vi "DAQ_connect.vi"(10 "thermocouple type":i32(ring)=10073 items=["J"=10072, "K"=10073, "N"=10077, "R"=10082, "S"=10085, "T"=10086, "B"=10047, "E"=10055], 11 "Array":tag[](array[tag])=["Mod2/ai1", "Mod2/ai2"]) -> (0 "error out":errorcluster, 3 "Refnum out":refnum<k21>)   [LabVIEW 2021, in "DAQ_Termopares.lvlib"]
uses:
  DAQ_Termopares.lvlib
  <vilib>/DAQmx/create/channels.llb/DAQmx Create Channel (AI-Temperature-Thermocouple).vi
panel:
  out "Array 2":errorcluster[](array[cluster])
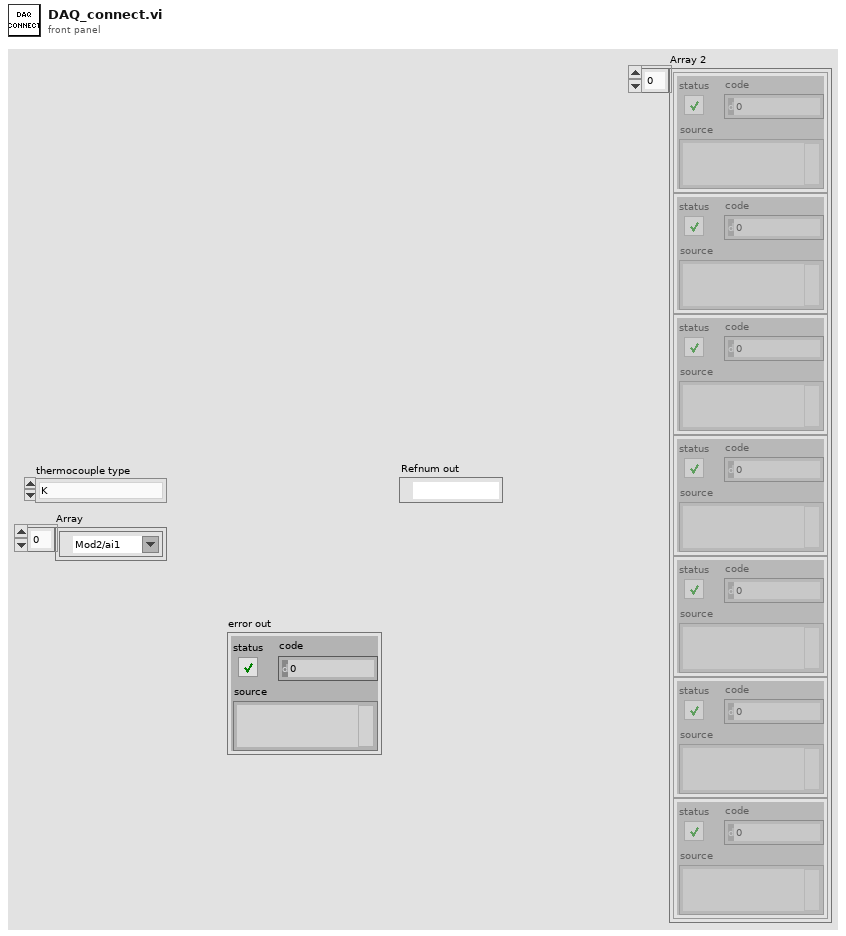
[diagram p1: front panel]
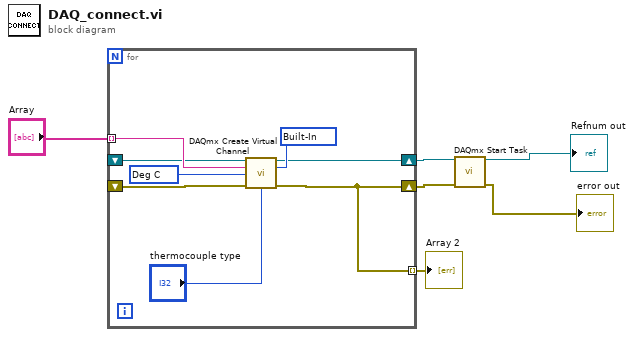
[diagram p0: block diagram]
diagram:
  n1 = for {
    tunnel: "Array" -> [w12] mode=indexing
    shift-right: [w7] -> w6
    shift-left: _ -> [w9]
    shift-right: [w11] -> w5
    shift-left: _ -> [w10]
    tunnel: [w7] -> w1 mode=indexing
    w14 = 10200 items=["Built-In"=10200, "Constant Value"=10116, "Channel"=10113] ("cjc source")
    w13 = 10143 items=["Deg C"=10143, "Deg F"=10144, "Kelvins"=10325, "Deg R"=10145, "From Custom Scale"=10065] ("units")
    n2 = call-poly <vilib>:"DAQmx Create Virtual Channel.vi"("task in"=w10, "physical channels"=w12, "cjc source"=w14, "units"=w13, "error in"=w9, "thermocouple type"="thermocouple type") -> ("task out"=w11:refnum<k21>, "error out"=w7:errorcluster)  [unwired: 8 in]
  }
  "Array 2" <- w1
  n3 = call <vilib>:"DAQmx Start Task.vi"("task/channels in"=w5, "error in"=w6) -> ("task out"=→"Refnum out":refnum<k21>, "error out"=→"error out":errorcluster)  [unwired: 12 in]
